vi "NP_Control.vi"(8 "error in (no error)":errorcluster, 9 "Color Box":u32(colorbox), 11 "VISA resource name":refnum<visa-resource-name>) -> (0 "error out":errorcluster, 3 "VISA resource name out":refnum<visa-resource-name>)   [LabVIEW 2025]
doc: "VI que permite utilizar las 3 Neo Pixel y asignarles un mismo color \nSe puede enviar el numero de 32 bits o usar la color box\nNo requiere input de pin ya que asume que se esta utilizando la placa Galiot de universidad Galileo"
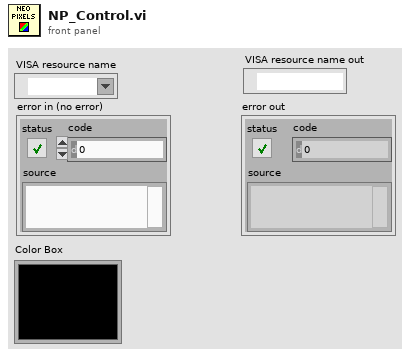
[diagram p1: front panel]
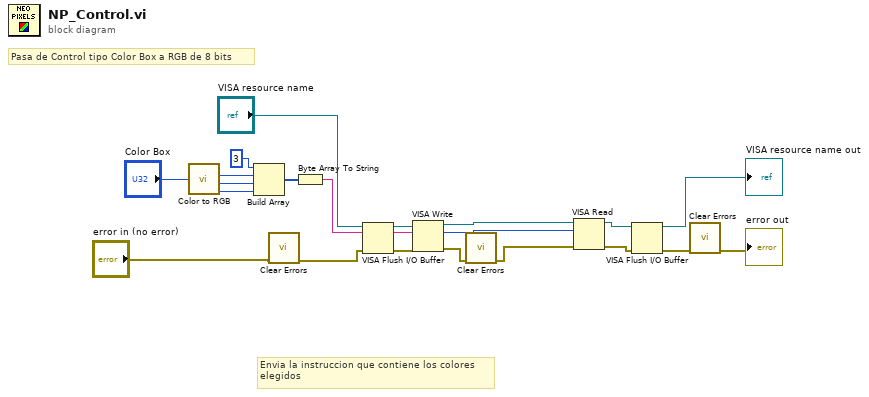
[diagram p0: block diagram]
diagram:
  # "Envia la instruccion que contiene los colores\nelegidos"
  # "Pasa de Control tipo Color Box a RGB de 8 bits"
  n1 = call <vilib>:"Color to RGB.vi"("Color"="Color Box") -> ("R"=w18:u8, "G"=w17:u8, "B"=w16:u8)  [unwired: 1 out]
  n2 = Build Array(u8 3 ("element"), w18, w17, w16) -> (w14:u8[])
  n3 = call <vilib>:"Clear Errors.vi"("error in (no error)"="error in (no error)") -> ("error out"=w2:errorcluster)  [unwired: 5 in, 1 out]
  n4 = Byte Array To String(unsigned byte array=w14) -> (string=w21:string)
  n5 = VISA Flush I/O Buffer(VISA resource name="VISA resource name", error in (no error)=w2) -> (VISA resource name out=w4:refnum<visa-resource-name>, error out=w3:errorcluster)  [unwired: 1 in]
  n6 = VISA Write(VISA resource name=w4, write buffer=w21, error in (no error)=w3) -> (VISA resource name out=w20:refnum<visa-resource-name>, return count=w13:u32, error out=w9:errorcluster)
  n7 = call <vilib>:"Clear Errors.vi"("error in (no error)"=w9) -> ("error out"=w10:errorcluster)  [unwired: 5 in, 1 out]
  n8 = VISA Read(VISA resource name=w20, byte count=w13, error in (no error)=w10) -> (VISA resource name out=w6:refnum<visa-resource-name>, error out=w8:errorcluster)  [unwired: 2 out]
  n9 = VISA Flush I/O Buffer(VISA resource name=w6, error in (no error)=w8) -> (VISA resource name out=→"VISA resource name out":refnum<visa-resource-name>, error out=w7:errorcluster)  [unwired: 1 in]
  n10 = call <vilib>:"Clear Errors.vi"("error in (no error)"=w7) -> ("error out"=→"error out":errorcluster)  [unwired: 5 in, 1 out]
